vi "Attitude Control Open.vi"(10 "Scene Graph":refnum<vi>) -> (0 "error out":errorcluster, 3 "Attitude Control Handle":T1)   [LabVIEW 2022 SP3, in "lv-attitudecontrol.lvlib"]
uses:
  lv-attitudecontrol.lvlib
  Controls/AttitudeHandle.ctl
  <vilib>/picture/3D Picture Control/NI_3D Picture Control.lvlib
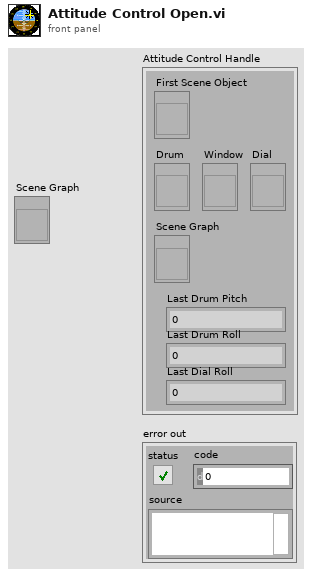
[diagram p1: front panel]
types:
  T1 = typedef "lv-attitudecontrol.lvlib/AttitudeHandle.ctl" = cluster{"First Scene Object":refnum<vi>, "Drum":refnum<vi>, "Window":refnum<vi>, "Dial":refnum<vi>, "Scene Graph":refnum<vi>, "Last Drum Pitch":dbl, "Last Drum Roll ":dbl, "Last Dial Roll":dbl}
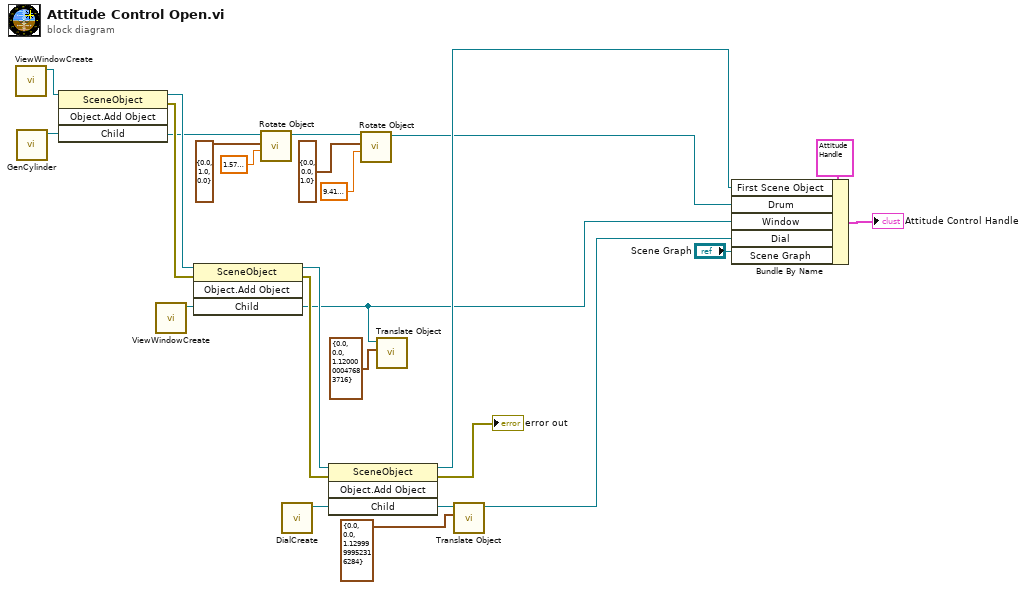
[diagram p0: block diagram]
diagram:
  n1 = call "ViewWindowCreate.vi"() -> ("SceneObject out"=w24:refnum<vi>)  [unwired: 11 in]
  n2 = call "GenCylinder.vi"() -> ("SceneObject out"=w10:refnum<vi>)  [unwired: 11 in]
  n3 = invoke class="SceneObject" method="Object.Add Object"(reference=w24, "Child"=w10) -> (reference out=w20:refnum<vi>, error out=w21:errorcluster, "Child"=w16:refnum<vi>)  [unwired: 2 in, 1 out]
  n4 = call "ViewWindowCreate.vi"() -> ("SceneObject out"=w25:refnum<vi>)  [unwired: 11 in]
  n5 = invoke class="SceneObject" method="Object.Add Object"(reference=w20, error in=w21, "Child"=w25) -> (reference out=w8:refnum<vi>, error out=w22:errorcluster, "Child"=w4:refnum<vi>)  [unwired: 1 in, 1 out]
  n6 = call <vilib>:"Rotate Object.vi"("Angle"=sgl 1.5799999 ("Angle 2"), "Axis"=cluster{"X":sgl, "Y":sgl, "Z":sgl} {"X"=0.0, "Y"=1.0, "Z"=0.0} ("Axis 2"), "Scene.Object In"=w16) -> ("Scene.Object Out"=w17:refnum<vi>)  [unwired: 7 in, 1 out]
  n7 = call "DialCreate.vi"() -> ("SceneObject out"=w9:refnum<vi>)  [unwired: 11 in]
  n8 = invoke class="SceneObject" method="Object.Add Object"(reference=w8, error in=w22, "Child"=w9) -> (reference out=w6:refnum<vi>, error out=→"error out":errorcluster, "Child"=w13:refnum<vi>)  [unwired: 1 in, 1 out]
  n9 = call <vilib>:"Rotate Object.vi"("Angle"=sgl 9.419999 ("Angle 3"), "Axis"=cluster{"X":sgl, "Y":sgl, "Z":sgl} {"X"=0.0, "Y"=0.0, "Z"=1.0} ("Axis 3"), "Scene.Object In"=w17) -> ("Scene.Object Out"=w5:refnum<vi>)  [unwired: 7 in, 1 out]
  n10 = call <vilib>:"Translate Object.vi"("Translation"=cluster{"X":sgl, "Y":sgl, "Z":sgl} {"X"=0.0, "Y"=0.0, "Z"=1.12} ("Translation 4"), "Scene.Object In"=w4) -> ()  [unwired: 8 in, 2 out]
  n11 = call <vilib>:"Translate Object.vi"("Translation"=cluster{"X":sgl, "Y":sgl, "Z":sgl} {"X"=0.0, "Y"=0.0, "Z"=1.13} ("Translation 5"), "Scene.Object In"=w13) -> ("Scene.Object Out"=w3:refnum<vi>)  [unwired: 8 in, 1 out]
  n12 = Bundle By Name(cluster=T1 {"First Scene Object"=refnum, "Drum"=refnum, "Window"=refnum, "Dial"=refnum, "Scene Graph"=refnum, "Last Drum Pitch"=0.0, "Last Drum Roll "=0.0, "Last Dial Roll"=0.0} ("Attitude Control Handle"), "First Scene Object"=w6, "Drum"=w5, "Window"=w4, "Dial"=w3, "Scene Graph"="Scene Graph") -> (→"Attitude Control Handle":T1)
